vi "IVI Error Converter.vi"(8 "error in (no error)":errorcluster {"code" format="%.0x"}, 10 "IVI error code (0)":i32 format="%.0x", 11 "instrument handle":u32) -> (0 "error out":errorcluster {"code" format="%.0x"}, 3 "instrument handle out":u32)   [LabVIEW 2009, in "Keysight XSAnVMA.lvlib"]
doc: "This VI converts error codes from IVI instrument drivers to standard LabVIEW error codes. If an error is detected the VI builds the appropriate error cluster that is readable by one of the error handlers supplied with LabVIEW."
uses:
  <instrlib>/Keysight XSAnVMA/Keysight XSAnVMA.lvlib
  KtXSAnVMA.dll
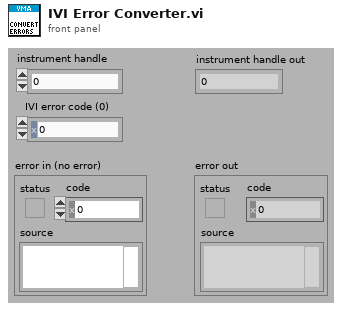
[diagram p1: front panel]
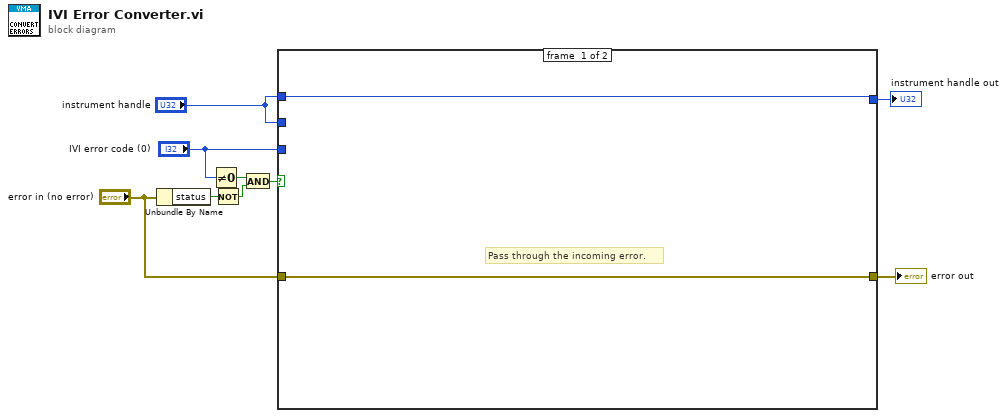
[diagram p0: block diagram]
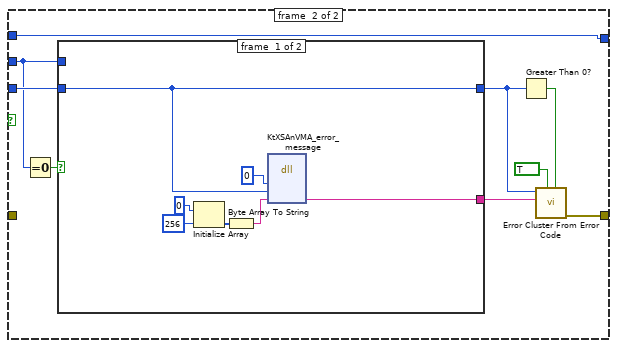
[diagram p2: hidden frame]
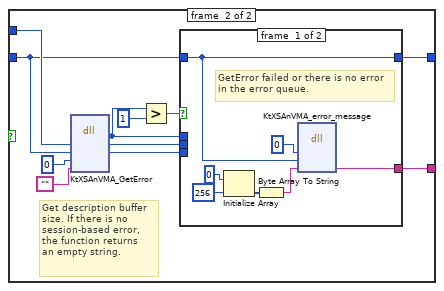
[diagram p3: hidden frame]
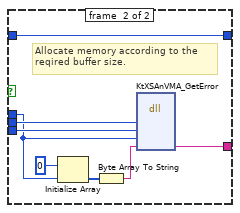
[diagram p4: hidden frame]
diagram:
  n1 = Unbundle By Name("error in (no error)") -> ("status"=w5:bool)
  n2 = Not Equal To 0?(x="IVI error code (0)") -> (x != 0?=w6:bool)
  n3 = Not(x=w5) -> (.not. x?=w4:bool)
  n4 = And(x=w6, y=w4) -> (x .and. y?=w3:bool)
  n5 = case shown="True" w3 {
    tunnel: "IVI error code (0)" -> [_ w20]
    tunnel: [w11 w15] -> w9
    tunnel: "instrument handle" -> [_ w13]
    tunnel: "error in (no error)" -> [w11 _]
    tunnel: [w10 w12] -> w2
    tunnel: "instrument handle" -> [w10 w12]
    frame #0 {
      # "Pass through the incoming error."
    }
    frame #1 {
      n6 = Equal To 0?(x=w13) -> (x = 0?=w14:bool)
      n7 = case shown="False" w14 {
        tunnel: w13 -> [_ w38]
        tunnel: w20 -> [w21 w30]
        tunnel: [w22 w29] -> w19
        tunnel: [w21 w28] -> w17
        frame #0 {
          n8 = Initialize Array(u8 0, 256) -> (w25:u8[])
          n9 = Byte Array To String(unsigned byte array=w25) -> (string=w27:string)
          n10 = dll-call lib="KtXSAnVMA**.dll" fn="KtXSAnVMA_error_message" label="error_message"("instrumentHandle"=0, "errorCode"=w21, "errorMessage"=w27) -> ("errorMessage"=w22:string)  [unwired: 5 in, 3 out]
        }
        frame #1 {
          # "Get description buffer\nsize. If there is no\nsession-based error,\nthe function returns\nan empty string."
          n11 = dll-call lib="KtXSAnVMA**.dll" fn="KtXSAnVMA_GetError" label="GetError"("vi"=w38, "errorCode"=w30, "bufferSize"=0, "description"="") -> (w33:i32, "vi"=w32:u32, "errorCode"=w31:i32)  [unwired: 4 in, 3 out]
          n12 = Greater?(x=w33, y=1) -> (0:w34:bool)
          n13 = case shown="True" w34 {
            tunnel: w33 -> [_ w49]
            tunnel: w32 -> [_ w53]
            tunnel: w31 -> [_ w52]
            tunnel: [w39 w47] -> w29
            tunnel: w30 -> [w40 w46]
            tunnel: [w40 w46] -> w28
            frame #0 {
              # "GetError failed or there is no error\nin the error queue."
              n14 = Initialize Array(u8 0, 256) -> (w43:u8[])
              n15 = Byte Array To String(unsigned byte array=w43) -> (string=w45:string)
              n16 = dll-call lib="KtXSAnVMA**.dll" fn="KtXSAnVMA_error_message" label="error_message"("instrumentHandle"=0, "errorCode"=w40, "errorMessage"=w45) -> ("errorMessage"=w39:string)  [unwired: 5 in, 3 out]
            }
            frame #1 {
              # "Allocate memory according to the\nreqired buffer size."
              n17 = Initialize Array(u8 0, w49) -> (w51:u8[])
              n18 = Byte Array To String(unsigned byte array=w51) -> (string=w48:string)
              n19 = dll-call lib="KtXSAnVMA**.dll" fn="KtXSAnVMA_GetError" label="GetError"("vi"=w53, "errorCode"=w52, "bufferSize"=w49, "description"=w48) -> ("description"=w47:string)  [unwired: 6 in, 3 out]
            }
          }
        }
      }
      n20 = Greater Than 0?(x=w17) -> (x > 0?=w16:bool)
      n21 = call <vilib>:"Error Cluster From Error Code.vi"("is warning? (False)"=w16, "show call chain? (False)"=TRUE, "error message (\"\")"=w19, "error code (0)"=w17) -> ("error out"=w15:errorcluster)  [unwired: 1 in, 4 out]
    }
  }
  "error out" <- w9
  "instrument handle out" <- w2
